vi "Modbus RTU Serial Simulator.vi"() -> ()   [LabVIEW 2014]
uses:
  <vilib>/Instr/_visa.llb/VISA Configure Serial Port (Instr).vi
panel:
  in  "列表框元素个数":i32=100
  in  "读寄存器请求":i32(listbox)
  in  "写寄存器请求":i32(listbox)
  out "error out":errorcluster caption="错误输出"
  in  "VISA resource name":refnum<visa-resource-name>="COM2" caption="VISA资源名称"
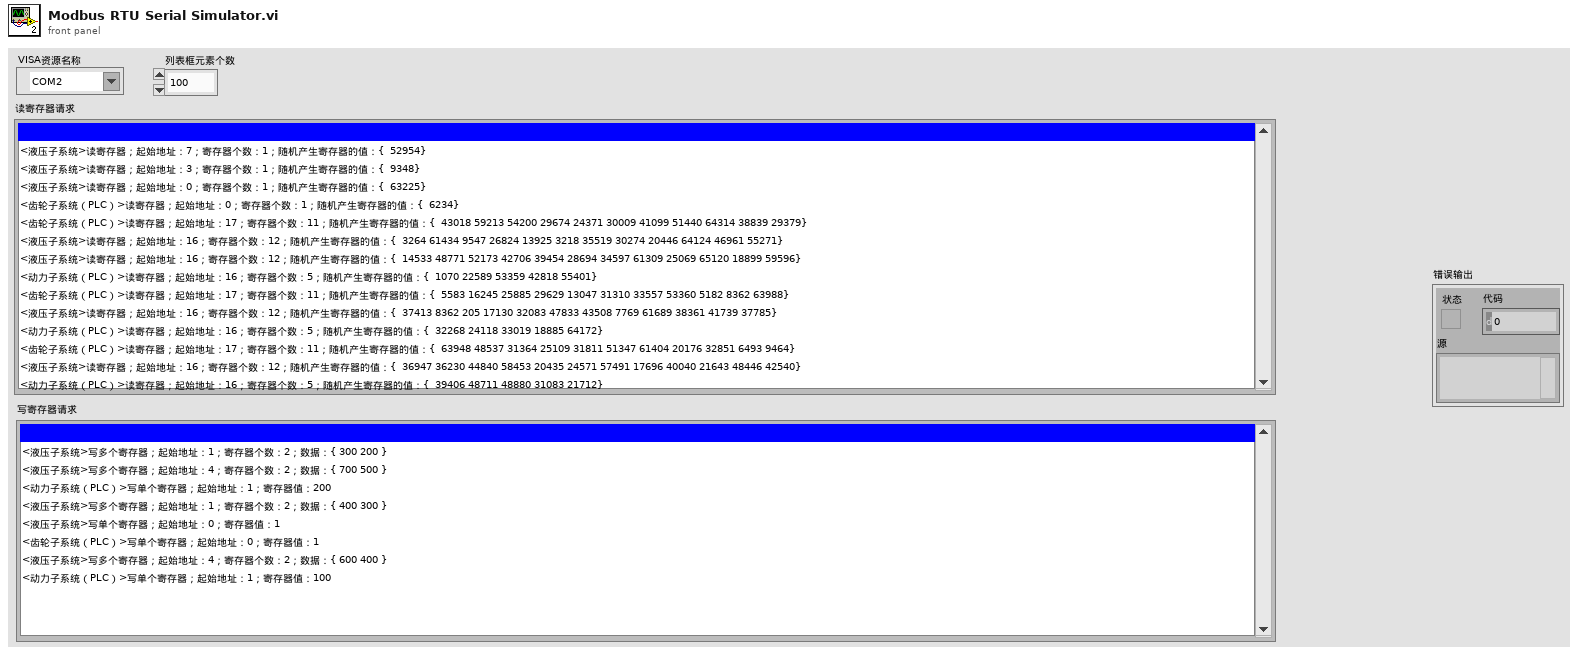
[diagram p1: front panel]
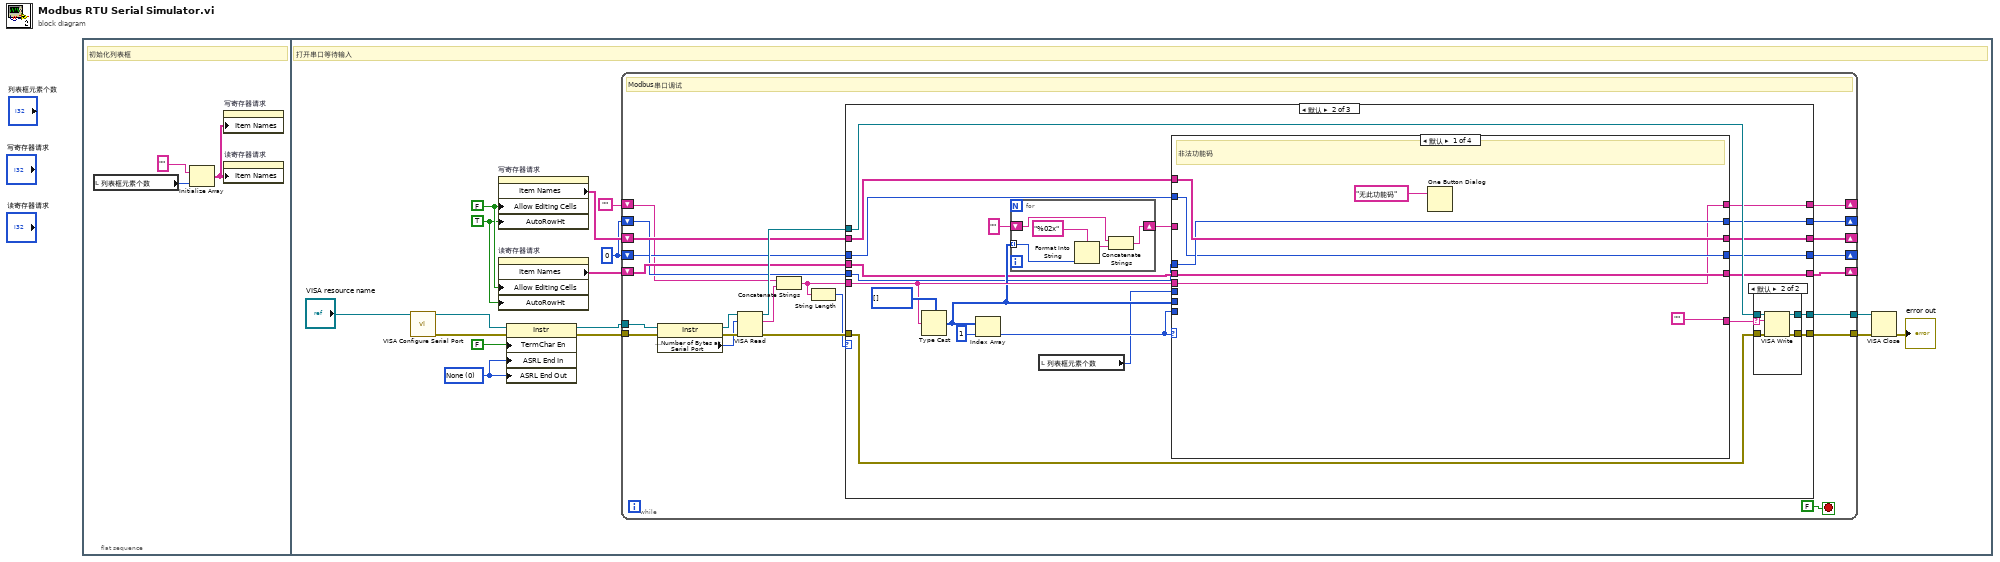
[diagram p0: block diagram]
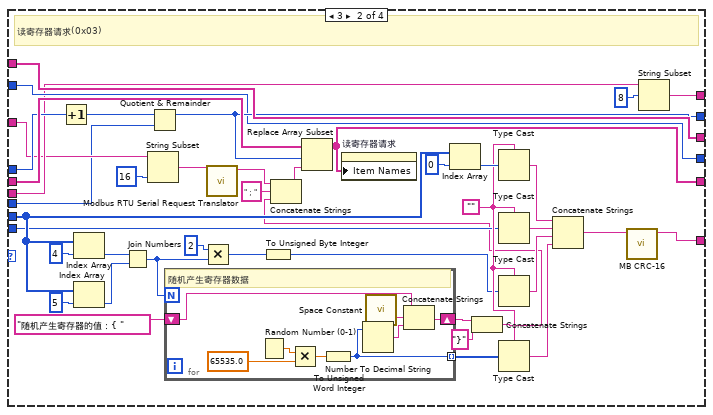
[diagram p4: hidden frame]
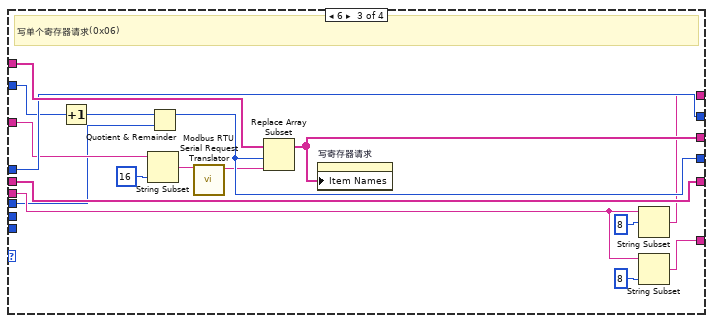
[diagram p5: hidden frame]
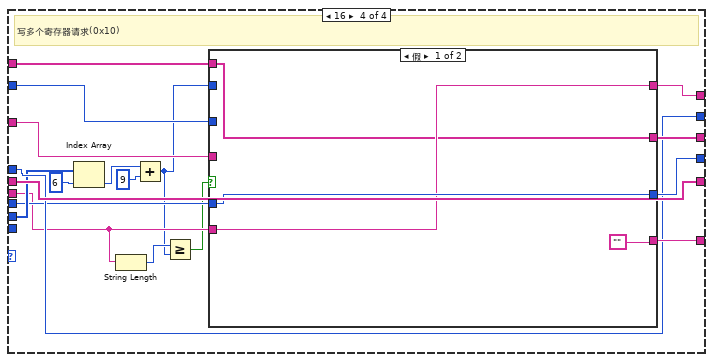
[diagram p6: hidden frame]
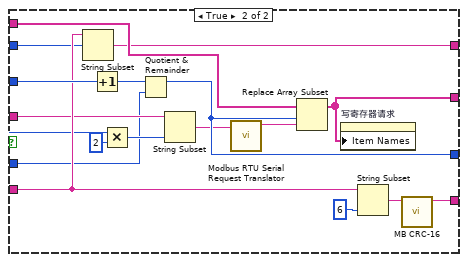
[diagram p7: hidden frame]
diagram:
  n1 = flat-sequence {
    frame #0 {
      # "初始化列表框"
      n2 = local read "列表框元素个数"() -> (w1:i32)
      n3 = Initialize Array("", w1) -> (w2:string[])
      n4 = property on="写寄存器请求" class="LstBox (严格)"("Item Names"=w2) -> ()  [unwired: 2 in, 2 out]
      n5 = property on="读寄存器请求" class="LstBox (严格)"("Item Names"=w2) -> ()  [unwired: 2 in, 2 out]
    }
    frame #1 {
      w5 = 0
      w7 = TRUE ("自动调整行高")
      w8 = FALSE ("允许编辑单元格")
      w10 = u16 0 items=["None", "Last Bit", "TermChar"] ("Serial Settings:End Mode for Reads")
      # "打开串口等待输入"
      n6 = call-poly "VISA Configure Serial Port"("VISA resource name"="VISA resource name") -> ("VISA resource name out"=w15:refnum<visa-resource-name>, "error out"=w14:errorcluster)  [unwired: 13 in]
      n7 = property on="写寄存器请求" class="LstBox (严格)"("Allow Editing Cells"=w8, "AutoRowHt"=w7) -> ("Item Names"=w9:string[])  [unwired: 2 in, 2 out]
      n8 = property on="读寄存器请求" class="LstBox (严格)"("Allow Editing Cells"=w8, "AutoRowHt"=w7) -> ("Item Names"=w6:string[])  [unwired: 2 in, 2 out]
      n9 = property class="Instr"(reference=w15, error in=w14, "TermChar En"=FALSE ("Message Based Settings:Send End Enable"), "ASRL End In"=w10, "ASRL End Out"=w10) -> (reference out=w13:refnum<visa-resource-name>, error out=w12:errorcluster)
      n10 = while {
        tunnel: w12 -> [w33]
        tunnel: [w42] -> w17
        tunnel: w13 -> [w34]
        tunnel: [w41] -> w18
        shift-right: [w31] -> _
        shift-left: w9 -> [w32]
        shift-right: [w30] -> _
        shift-left: w6 -> [w29]
        shift-right: [w25] -> _
        shift-left: w5 -> [w28]
        shift-right: [w26] -> _
        shift-left: w5 -> [w27]
        shift-right: [w22] -> _
        shift-left: "" -> [w24]
        stop <- FALSE stop-if-true
        # "Modbus串口调试"
        n11 = property class="Instr"(reference=w34, error in=w33) -> (reference out=w38:refnum<visa-resource-name>, error out=w37:errorcluster, "Serial Settings:Number of Bytes at Serial Port"=w36:u32)
        n12 = VISA Read(VISA resource name=w38, byte count=w36, error in (no error)=w37) -> (VISA resource name out=w39:refnum<visa-resource-name>, read buffer=w23:string, error out=w35:errorcluster)  [unwired: 1 out]
        n13 = Concatenate Strings(w24, w23) -> (w21:string)
        n14 = String Length(string=w21) -> (length=w20:i32)
        n15 = case shown="默认" w20 {
          tunnel: [w48 w66 w201] -> w42
          tunnel: [w47 w67 w202] -> w41
          tunnel: w39 -> [w47 w69 w202]
          tunnel: w35 -> [w48 w68 w201]
          tunnel: w21 -> [w49 w64 w196]
          tunnel: w32 -> [w45 w60 w200]
          tunnel: [w45 w59 w200] -> w31
          tunnel: [w43 w58 w199] -> w30
          tunnel: w29 -> [w43 w57 w199]
          tunnel: w28 -> [w44 w56 w198]
          tunnel: w27 -> [w46 w55 w197]
          tunnel: [w46 w54 w197] -> w26
          tunnel: [w44 w53 w198] -> w25
          tunnel: [w49 w52 w196] -> w22
          frame 1..7 {
          }
          frame Default {
            n16 = Type Cast(type=u8[] [], x=w64) -> (*(type *) &x=w63:u8[])
            n17 = Index Array(array=w63, index=1 ("索引")) -> (element=w65:u8)
            n18 = for {
              tunnel: w63 -> [w83] mode=indexing
              shift-right: [w79] -> w61
              shift-left: "" -> [w80]
              n19 = Format Into String(format string="%02x" ("格式字符串"), w83) -> (resulting string=w81:string)  [unwired: 2 in, 1 out]
              n20 = Concatenate Strings(w80, w81) -> (w79:string)
            }
            n21 = local read "列表框元素个数"() -> (w51:i32)
            n22 = case shown="默认" w65 {
              tunnel: w65 -> [_ w105 _ _]
              tunnel: ["" w123 w146 w174] -> w50
              tunnel: w63 -> [_ w106 _ w167]
              tunnel: w64 -> [w85 w104 w147 w160]
              tunnel: w61 -> [_ w102 w144 w162]
              tunnel: w60 -> [w89 w111 w156 w173]
              tunnel: [w89 w111 w155 w171] -> w59
              tunnel: [w88 w113 w154 w172] -> w58
              tunnel: w57 -> [w88 w112 w154 w172]
              tunnel: w56 -> [w87 w107 w153 w168]
              tunnel: w55 -> [w86 w108 w151 w170]
              tunnel: [w86 w108 w150 w169] -> w54
              tunnel: [w87 w109 w153 w168] -> w53
              tunnel: [w85 w103 w148 w163] -> w52
              tunnel: w51 -> [_ w99 w142 w161]
              frame Default {
                # "非法功能码"
                n23 = One Button Dialog(message="无此功能码" ("消息")) -> ()  [unwired: 1 in, 1 out]
              }
              frame 3 {
                w126 = ""
                # "读寄存器请求(0x03)"
                n24 = Increment(x=w107) -> (x+1=w110:i32)
                n25 = Index Array(array=w106, index=4 ("索引")) -> (element=w120:u8)
                n26 = Index Array(array=w106, index=5 ("索引")) -> (element=w119:u8)
                n27 = Join Numbers(hi=w120, lo=w119) -> ((hi.lo)=w115:u16)
                n28 = String Subset(string=w102, length (rest)=16 ("长度（剩余）")) -> (substring=w98:string)  [unwired: 1 in]
                n29 = Quotient & Remainder(x=w110, y=w99) -> (x-y*floor(x/y)=w109:i32)  [unwired: 1 out]
                n30 = for {
                  N: w115 -> [_]
                  tunnel: [w136] -> w114 mode=indexing
                  shift-right: [w132] -> w96
                  shift-left: "随机产生寄存器的值：{ " -> [w135]
                  # "随机产生寄存器数据"
                  n31 = Random Number (0-1)() -> (number: 0 to 1=w139:dbl)
                  n32 = Multiply(x=w139, y=65535.0) -> (x*y=w137:dbl)
                  n33 = To Unsigned Word Integer(number=w137) -> (unsigned 16bit integer=w136:u16)
                  n34 = Number To Decimal String(number=w136) -> (decimal integer string=w133:string)  [unwired: 1 in]
                  n35 = call <vilib>:"Space Constant.vi"() -> ("String"=w134:string)
                  n36 = Concatenate Strings(w135, w134, w133) -> (w132:string)
                }
                n37 = Multiply(x=u16 2, y=w115) -> (x*y=w117:u16)
                n38 = call "Modbus RTU Serial Request Translator.vi"("请求字符串"=w98) -> ("转换后的字符串"=w93:string)  [unwired: 10 in]
                n39 = To Unsigned Byte Integer(number=w117) -> (unsigned 8bit integer=w116:u8)
                n40 = Index Array(array=w106, index=0 ("索引")) -> (element=w130:u8)
                n41 = Concatenate Strings(w96, "}" ("字符串")) -> (w92:string)
                n42 = Concatenate Strings(w93, "；" ("字符串"), w92) -> (w91:string)
                n43 = Replace Array Subset(array=w112, new element=w91, index=w109) -> (w113:string[])
                n44 = property on="读寄存器请求" class="LstBox (严格)"("Item Names"=w113) -> ()  [unwired: 2 in, 2 out]
                n45 = Type Cast(type=w126, x=w130) -> (*(type *) &x=w129:string)
                n46 = Type Cast(type=w126, x=w105) -> (*(type *) &x=w128:string)
                n47 = Type Cast(type=w126, x=w116) -> (*(type *) &x=w127:string)
                n48 = Type Cast(type=w126, x=w114) -> (*(type *) &x=w125:string)
                n49 = Concatenate Strings(w129, w128, w127, w125) -> (w124:string)
                n50 = call "MB CRC-16.vi"("String"=w124) -> ("String & CRC-16"=w123:string)  [unwired: 8 in, 2 out]
                n51 = String Subset(string=w104, offset (0)=8 ("偏移量(0)")) -> (substring=w103:string)  [unwired: 1 in]
              }
              frame 6 {
                # "写单个寄存器请求(0x06)"
                n52 = Increment(x=w151) -> (x+1=w152:i32)
                n53 = String Subset(string=w144, length (rest)=16 ("长度（剩余）")) -> (substring=w141:string)  [unwired: 1 in]
                n54 = Quotient & Remainder(x=w152, y=w142) -> (x-y*floor(x/y)=w150:i32)  [unwired: 1 out]
                n55 = call "Modbus RTU Serial Request Translator.vi"("请求字符串"=w141) -> ("转换后的字符串"=w140:string)  [unwired: 10 in]
                n56 = Replace Array Subset(array=w156, new element=w140, index=w150) -> (w155:string[])
                n57 = property on="写寄存器请求" class="LstBox (严格)"("Item Names"=w155) -> ()  [unwired: 2 in, 2 out]
                n58 = String Subset(string=w147, offset (0)=8 ("偏移量(0)")) -> (substring=w148:string)  [unwired: 1 in]
                n59 = String Subset(string=w147, length (rest)=8 ("长度（剩余）")) -> (substring=w146:string)  [unwired: 1 in]
              }
              frame 16 {
                # "写多个寄存器请求(0x10)"
                n60 = Index Array(array=w167, index=6 ("索引")) -> (element=w165:u8)
                n61 = String Length(string=w160) -> (length=w159:i32)
                n62 = Add(x=w165, y=u8 9) -> (x+y=w158:u8)
                n63 = Greater Or Equal?(x=w159, y=w158) -> (x >= y?=w157:bool)
                n64 = case shown="假" w157 {
                  tunnel: ["" w193] -> w174
                  tunnel: w173 -> [w175 w192]
                  tunnel: [w175 w191] -> w171
                  tunnel: w170 -> [_ w190]
                  tunnel: [w177 w188] -> w169
                  tunnel: w160 -> [w176 w187]
                  tunnel: [w176 w186] -> w163
                  tunnel: w162 -> [_ w185]
                  tunnel: w158 -> [_ w184]
                  tunnel: w161 -> [w177 w181]
                  frame False {
                  }
                  frame True {
                    n65 = String Subset(string=w187, offset (0)=w184) -> (substring=w186:string)  [unwired: 1 in]
                    n66 = Increment(x=w190) -> (x+1=w189:i32)
                    n67 = Multiply(x=w184, y=u8 2) -> (x*y=w183:u8)
                    n68 = Quotient & Remainder(x=w189, y=w181) -> (x-y*floor(x/y)=w188:i32)  [unwired: 1 out]
                    n69 = String Subset(string=w185, length (rest)=w183) -> (substring=w180:string)  [unwired: 1 in]
                    n70 = call "Modbus RTU Serial Request Translator.vi"("请求字符串"=w180) -> ("转换后的字符串"=w179:string)  [unwired: 10 in]
                    n71 = Replace Array Subset(array=w192, new element=w179, index=w188) -> (w191:string[])
                    n72 = property on="写寄存器请求" class="LstBox (严格)"("Item Names"=w191) -> ()  [unwired: 2 in, 2 out]
                    n73 = String Subset(string=w187, length (rest)=6 ("长度（剩余）")) -> (substring=w194:string)  [unwired: 1 in]
                    n74 = call "MB CRC-16.vi"("String"=w194) -> ("String & CRC-16"=w193:string)  [unwired: 8 in, 2 out]
                  }
                }
              }
            }
            n75 = case shown="默认" w50 {
              selector: w50 -> [_ w74]
              tunnel: w69 -> [w73 w78]
              tunnel: w68 -> [w72 w77]
              tunnel: [w73 w76] -> w67
              tunnel: [w72 w75] -> w66
              frame "" {
              }
              frame Default {
                n76 = VISA Write(VISA resource name=w78, write buffer=w74, error in (no error)=w77) -> (VISA resource name out=w76:refnum<visa-resource-name>, error out=w75:errorcluster)  [unwired: 1 out]
              }
            }
          }
          frame 0 {
          }
        }
      }
      n77 = VISA Close(VISA resource name=w18, error in (no error)=w17) -> (error out=→"error out":errorcluster)
    }
  }
